vi "Adam_Ch_Control.vi"(1 "Turn On?":bool, 2 "ADAM Ch Names":string[](array[string])=["EnFlo Tun:Ultrasonic:Fixed"]) -> ()   [LabVIEW 2011]
uses:
  ADAM Controls/Channel_State.ctl
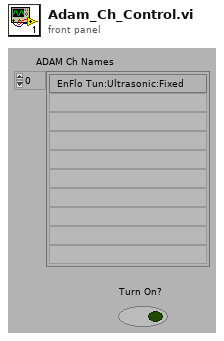
[diagram p1: front panel]
types:
  T1 = typedef "Channel_State.ctl" = enum16{"On", "Off", "Always On", "Always Off"}
  T2 = typedef "Ch_description_ADAM.ctl" = cluster{"Ch Name":string, "Type":T3, "Function":T4, "Ch State":T1, "Calibration type":T5, "A":dbl, "B":dbl, "C":dbl, "D":dbl, "Comments":string, "Address":T6, "String":string, "Duty":u16}
  T3 = typedef "Module_type_ADAM.ctl" = string
  T4 = typedef "Function_ADAM.ctl" = enum16{"Analogue Input", "Digital Input", "Event counter", "Event rate", "Analogue Output", "Digital Output", "Relay Output"}
  T5 = typedef "Calib_type_ADAM.ctl" = enum16{"Raw", "Bx + A", "Cx^2 + Bx + A", "Dx^3 + Cx^2 + Bx + A", "In Band", "Hi-Tec Q", "Hi-Tec M_dot", "Text"}
  T6 = typedef "Address.ctl" = cluster{"Main":i32, "Ch.":i32, "Sub":i32, "Port Name":string}
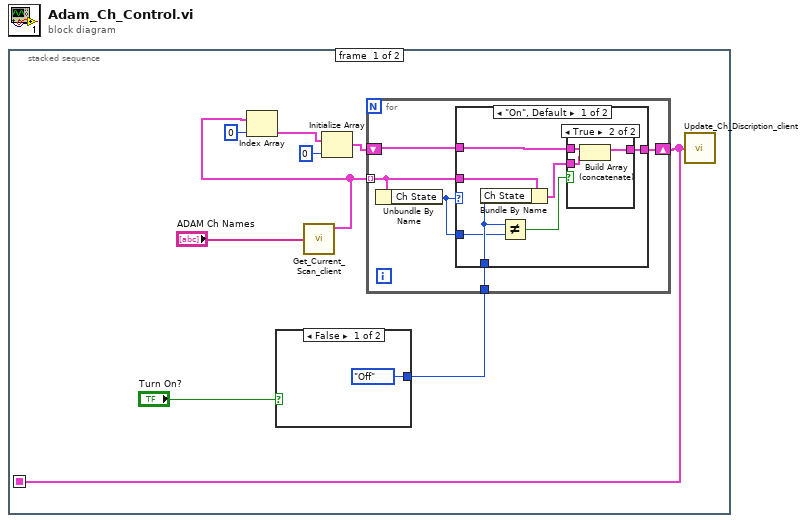
[diagram p0: block diagram]
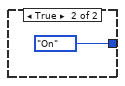
[diagram p2: hidden frame]
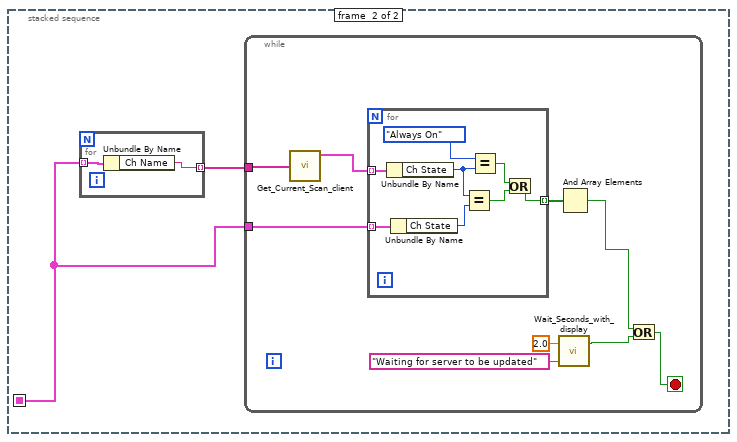
[diagram p5: hidden frame]
diagram:
  n1 = stacked-sequence {
    seq-local: [w3 _] -> [_ w29]
    frame #0 {
      n2 = case shown="False" "Turn On?" {
        tunnel: [Channel_State."Off" ("Ch State") Channel_State."On" ("Ch State")] -> w9
        frame False {
        }
        frame True {
        }
      }
      n3 = call "Get_Current_Scan_client.vi"("ADAM Ch Names"="ADAM Ch Names") -> ("Ch Description Array"=w5:T2[])  [unwired: 3 out]
      n4 = Index Array(array=w5, index=0) -> (element=w4:T2)
      n5 = Initialize Array(w4, 0 ("dimension size")) -> (w8:T2[])
      n6 = for {
        tunnel: w5 -> [w16] mode=indexing
        shift-right: [w13] -> w3
        shift-left: w8 -> [w14]
        tunnel: w9 -> [w15]
        n7 = Unbundle By Name(w16) -> ("Ch State"=w12:T1)
        n8 = case shown="\"On\", Default" w12 {
          tunnel: w16 -> [w23 _]
          tunnel: w15 -> [w19 _]
          tunnel: w14 -> [w22 w28]
          tunnel: [w20 w28] -> w13
          tunnel: w12 -> [w18 _]
          frame "On", Default {
            n9 = Bundle By Name(cluster=w23, "Ch State"=w19) -> (w21:T2)
            n10 = Not Equal?(x=w19, y=w18) -> (x != y?=w17:bool)
            n11 = case shown="True" w17 {
              tunnel: w22 -> [w24 w27]
              tunnel: w21 -> [_ w26]
              tunnel: [w24 w25] -> w20
              frame False {
              }
              frame True {
                n12 = Build Array (concatenate)(w27, w26) -> (w25:T2[])
              }
            }
          }
          frame "Always On" {
          }
        }
      }
      n13 = call "Update_Ch_Discription_client.vi"("Channels to update In"=w3) -> ()  [unwired: 1 out]
    }
    frame #1 {
      n14 = for {
        tunnel: w29 -> [w49] mode=indexing
        tunnel: [w48] -> w30 mode=indexing
        n15 = Unbundle By Name(w49) -> ("Ch Name"=w48:string)
      }
      n16 = while {
        tunnel: w30 -> [w39]
        tunnel: w29 -> [w37]
        stop <- w33 stop-if-true
        n17 = call "Get_Current_Scan_client.vi"("ADAM Ch Names"=w39) -> ("Ch Description Array"=w38:T2[])  [unwired: 3 out]
        n18 = for {
          tunnel: w38 -> [w47] mode=indexing
          tunnel: w37 -> [w46] mode=indexing
          tunnel: [w40] -> w36 mode=indexing
          n19 = Unbundle By Name(w47) -> ("Ch State"=w43:T1)
          n20 = Unbundle By Name(w46) -> ("Ch State"=w45:T1)
          n21 = Equal?(x=w43, y=w45) -> (x = y?=w42:bool)
          n22 = Equal?(x=Channel_State."Always On" ("Ch State"), y=w43) -> (x = y?=w41:bool)
          n23 = Or(x=w41, y=w42) -> (x .or. y?=w40:bool)
        }
        n24 = call "Wait_Seconds_with_display.vi"("Message"="Waiting for server to be updated", "Seconds to wait"=2.0) -> ("Stopped"=w34:bool)  [unwired: 1 out]
        n25 = And Array Elements(Boolean array=w36) -> (logical AND=w35:bool)
        n26 = Or(x=w35, y=w34) -> (x .or. y?=w33:bool)
      }
    }
  }
